vi "Login.vi"(9 "connection reference":T1, 10 "ACCOUNT:":string, 11 "Permission":string[](array[string])) -> (2 "OK":bool=TRUE, 3 "ACCOUNT:  2":string)   [LabVIEW 2015]
uses:
  <vilib>/addons/database/Connection.llb/Conn ObjectReference.ctl
  <vilib>/addons/database/_DB Variant To Data/Database Variant To Data.xnode
  <vilib>/addons/database/NI_Database_API.lvlib
  <vilib>/addons/database/Connection.llb/DB Tools Open Connec (String).vi
panel:
  out "Account Data":string[][](array[string])
  in  "Cancel":bool
  in  "Login":bool
  in  "PASSWORD:":string
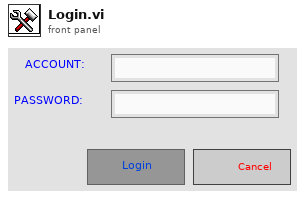
[diagram p1: front panel]
types:
  T1 = typedef "NI_Database_API.lvlib/Conn ObjectReference.ctl" = refnum<k1>
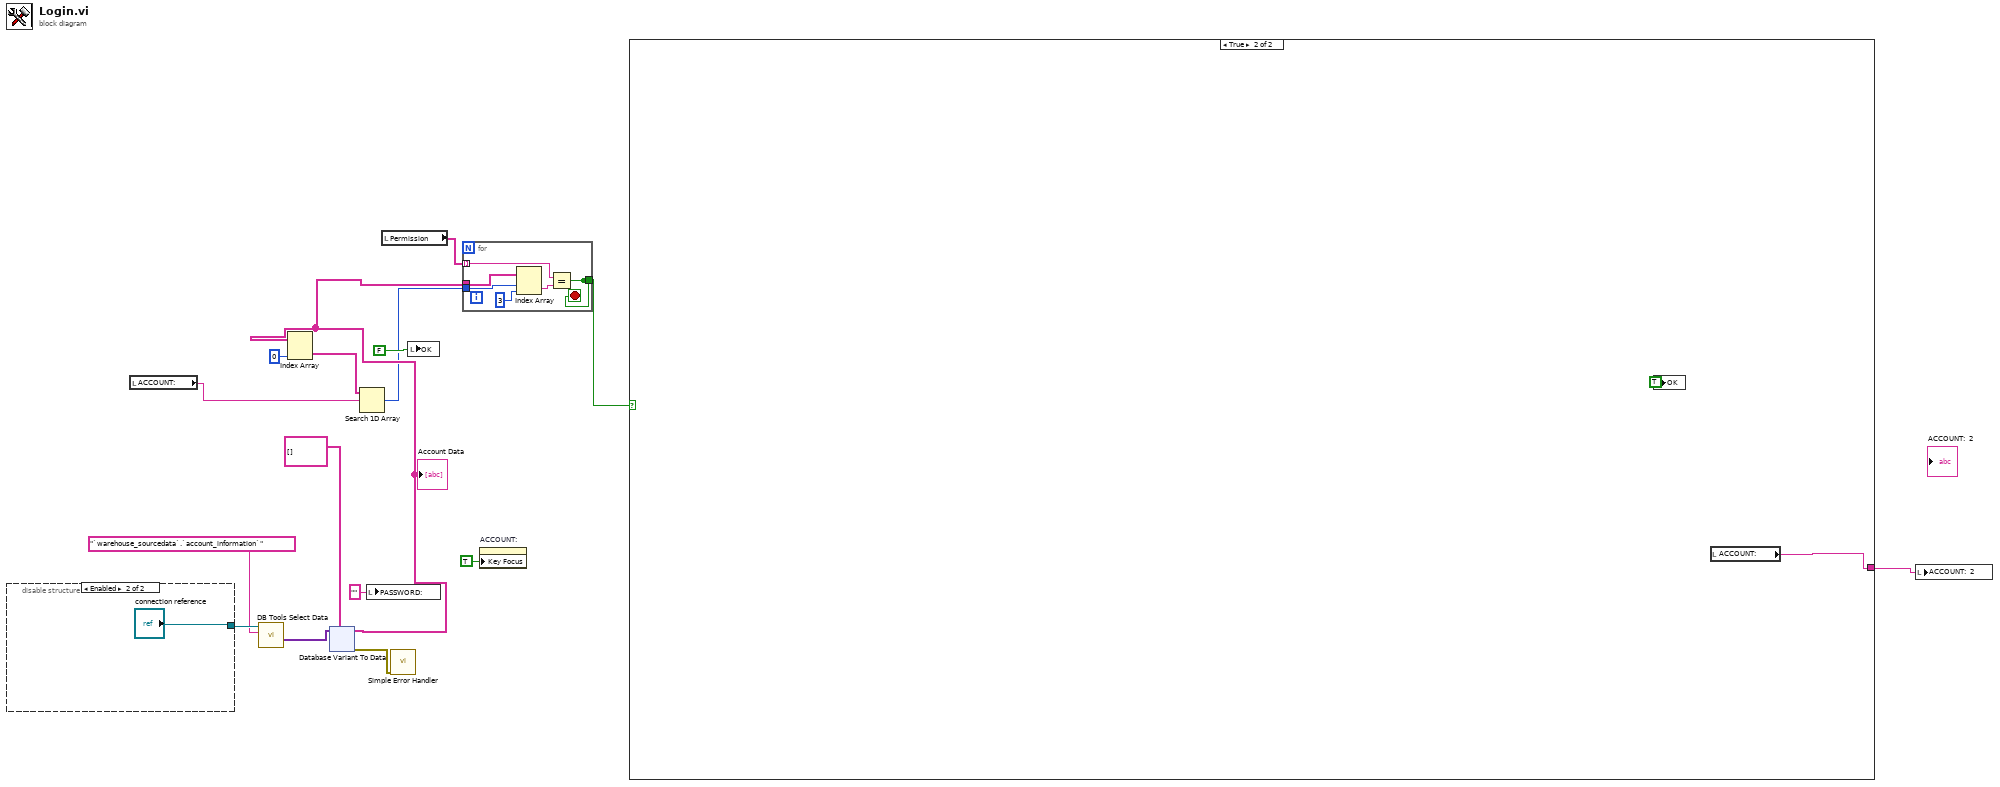
[diagram p0: block diagram]
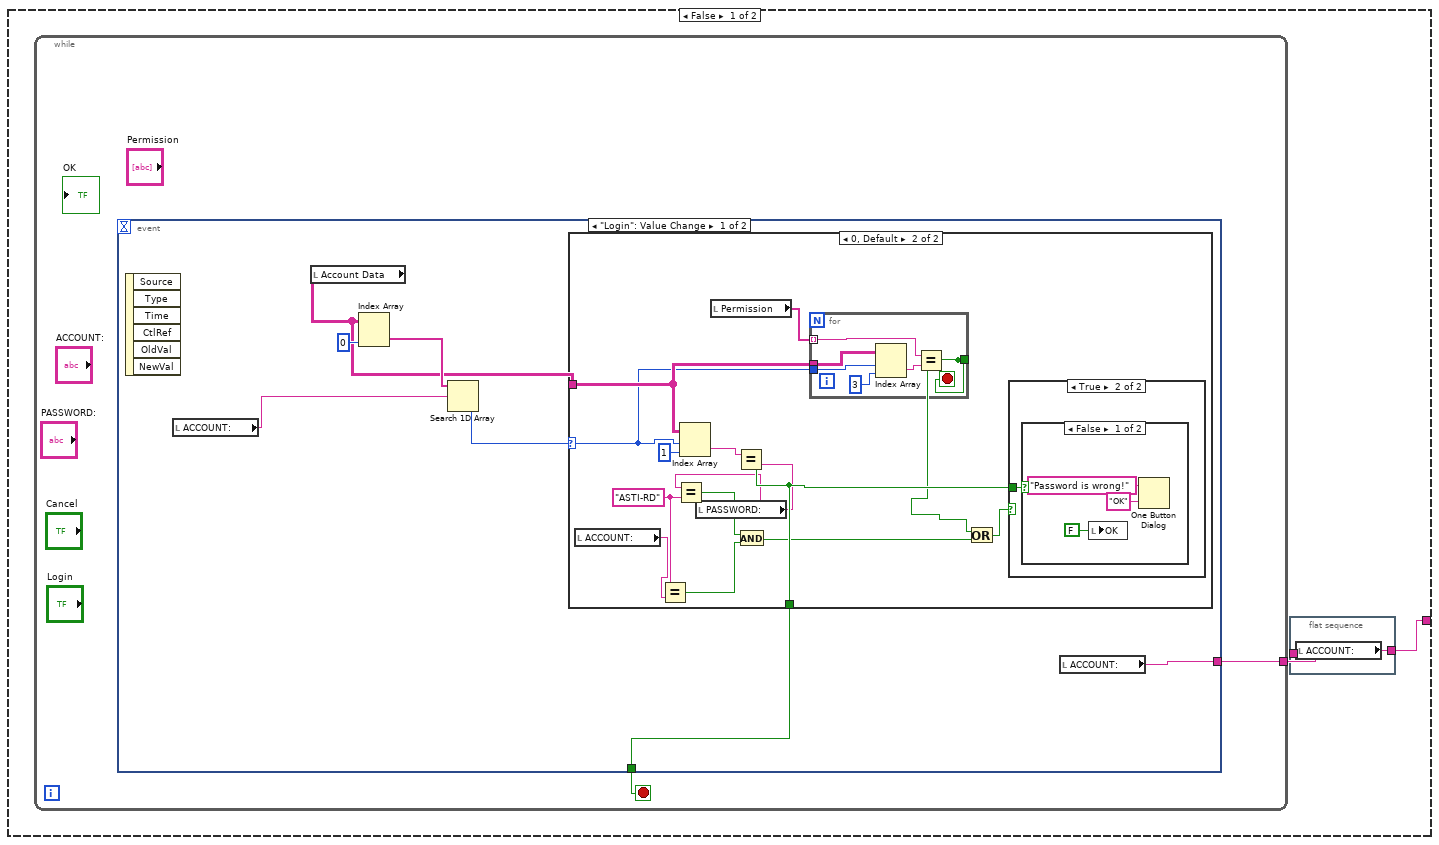
[diagram p2: hidden frame]
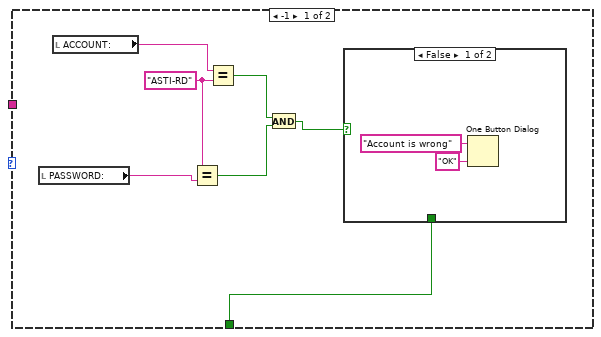
[diagram p3: hidden frame]
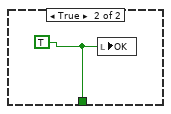
[diagram p4: hidden frame]
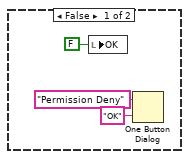
[diagram p5: hidden frame]
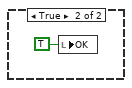
[diagram p6: hidden frame]
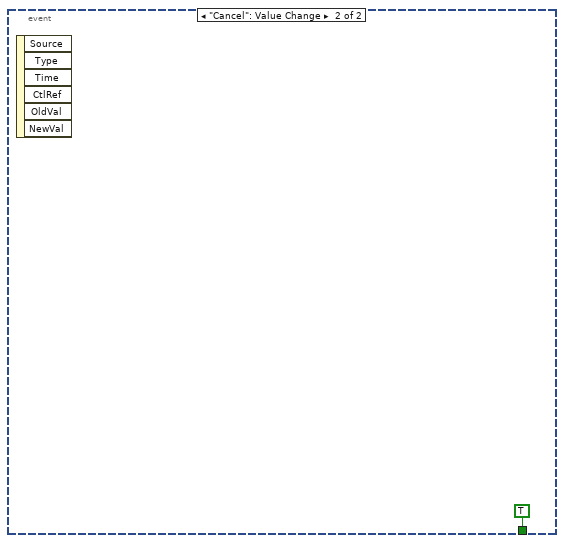
[diagram p7: hidden frame]
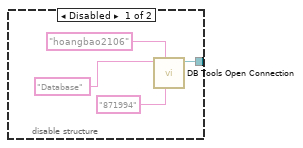
[diagram p8: hidden frame]
diagram:
  n1 = disable-structure shown="Enabled" {
    disable-tunnel: [w17 "connection reference"] -> w14
    frame Disabled {
      n2 = call-poly <vilib>:"DB Tools Open Connection.vi"("password"="871994" ("userID"), "userID"="hoangbao2106", "connection information"="Database" ("userID")) -> ("connection reference"=w17:T1)  [unwired: 5 in, 1 out]
    }
    frame Enabled {
    }
  }
  n3 = local read "ACCOUNT:"() -> (w7:string)
  n4 = call <vilib>:"DB Tools Select Data.vi"("table"="`warehouse_sourcedata`.`account_information`" ("userID"), "connection reference"=w14) -> ("data"=w12:variant[][])  [unwired: 4 in, 2 out]
  n5 = xnode "Database Variant To Data"("database variant"=w12, "type"=string[][] []) -> ("data"=w5:string[][], "error out"=w10:errorcluster)  [unwired: 1 in]
  "Account Data" <- w5
  n6 = Index Array(array=w5, index (col)=0 ("disabled index (col)")) -> (element=w9:string[])  [unwired: 1 in]
  n7 = Search 1D Array(1D array=w9, element=w7) -> (index of element=w4:i32)  [unwired: 1 in]
  n8 = local write "PASSWORD:"("" ("PASSWORD:")) -> ()
  n9 = local read "Permission"() -> (w6:string[])
  n10 = call <vilib>:"Simple Error Handler.vi"("error in (no error)"=w10) -> ()  [unwired: 4 in, 5 out]
  n11 = local write "OK"(FALSE) -> ()
  n12 = for {
    tunnel: w5 -> [w27]
    tunnel: w4 -> [w25]
    tunnel: w6 -> [w23] mode=indexing
    tunnel: [w22] -> w3
    stop <- w22 stop-if-true
    n13 = Index Array(array=w27, index (row)=w25, index (col)=3 ("index")) -> (element=w24:string)
    n14 = Equal?(x=w23, y=w24) -> (x = y?=w22:bool)
  }
  n15 = property on="ACCOUNT:" class="Str"("Key Focus"=TRUE) -> ()  [unwired: 2 in, 2 out]
  n16 = case shown="True" w3 {
    tunnel: [w28 w79] -> w2
    frame False {
      n17 = while {
        tunnel: [w31] -> w29
        stop <- w32 stop-if-true
        n18 = event shown="[0] \"Login\": Value Change" {
          selector: _ -> [_ _]
          dyn-events: _ -> [_ _]
          timeout: _ -> [_ _]
          tunnel: [w36 TRUE] -> w32
          tunnel: [w33 _] -> w31
          event "Login": Value Change {
            n19 = event-data() -> ()  [unwired: 1 in, 6 out]
            n20 = local read "ACCOUNT:"() -> (w37:string)
            n21 = local read "Account Data"() -> (w34:string[][])
            n22 = Index Array(array=w34, index (col)=0 ("disabled index (col)")) -> (element=w38:string[])  [unwired: 1 in]
            n23 = Search 1D Array(1D array=w38, element=w37) -> (index of element=w35:i32)  [unwired: 1 in]
            n24 = case shown="0, Default" w35 {
              selector: w35 -> [_ w58]
              tunnel: w34 -> [_ w59]
              tunnel: [w40 w60] -> w36
              frame -1 {
                w44 = "ASTI-RD" ("y")
                n25 = local read "PASSWORD:"() -> (w45:string)
                n26 = local read "ACCOUNT:"() -> (w46:string)
                n27 = Equal?(x=w44, y=w45) -> (x = y?=w42:bool)
                n28 = Equal?(x=w46, y=w44) -> (x = y?=w43:bool)
                n29 = And(x=w43, y=w42) -> (x .and. y?=w41:bool)
                n30 = case shown="False" w41 {
                  tunnel: [_ w49] -> w40
                  frame False {
                    n31 = One Button Dialog(message="Account is wrong", button name ("OK")="OK") -> ()  [unwired: 1 out]
                  }
                  frame True {
                    w49 = TRUE
                    n32 = local write "OK"(w49) -> ()
                  }
                }
              }
              frame 0, Default {
                w57 = "ASTI-RD" ("y")
                n33 = local read "ACCOUNT:"() -> (w51:string)
                n34 = Equal?(x=w57, y=w51) -> (x = y?=w55:bool)
                n35 = Index Array(array=w59, index (row)=w58, index (col)=1 ("disabled index (col)")) -> (element=w62:string)
                n36 = local read "PASSWORD:"() -> (w52:string)
                n37 = Equal?(x=w52, y=w57) -> (x = y?=w56:bool)
                n38 = local read "Permission"() -> (w61:string[])
                n39 = Equal?(x=w62, y=w52) -> (x = y?=w60:bool)
                n40 = And(x=w56, y=w55) -> (x .and. y?=w54:bool)
                n41 = for {
                  tunnel: w59 -> [w69]
                  tunnel: w58 -> [w67]
                  tunnel: w61 -> [w65] mode=indexing
                  tunnel: [w64] -> w50
                  stop <- w64 stop-if-true
                  n42 = Index Array(array=w69, index (row)=w67, index (col)=3 ("index")) -> (element=w66:string)
                  n43 = Equal?(x=w65, y=w66) -> (x = y?=w64:bool)
                }
                n44 = Or(x=w50, y=w54) -> (x .or. y?=w53:bool)
                n45 = case shown="True" w53 {
                  tunnel: w60 -> [_ w73]
                  frame False {
                    n46 = local write "OK"(FALSE ("OK")) -> ()
                    n47 = One Button Dialog(message="Permission Deny", button name ("OK")="OK") -> ()  [unwired: 1 out]
                  }
                  frame True {
                    n48 = case shown="False" w73 {
                      frame False {
                        n49 = local write "OK"(FALSE ("OK")) -> ()
                        n50 = One Button Dialog(message="Password is wrong!", button name ("OK")="OK") -> ()  [unwired: 1 out]
                      }
                      frame True {
                        n51 = local write "OK"(TRUE ("OK")) -> ()
                      }
                    }
                  }
                }
              }
            }
            n52 = local read "ACCOUNT:"() -> (w33:string)
          }
          event "Cancel": Value Change {
            n53 = event-data() -> ()  [unwired: 1 in, 6 out]
          }
        }
      }
      n54 = flat-sequence {
        tunnel: w29 -> [_]
        tunnel: [w30] -> w28
        frame #0 {
          n55 = local read "ACCOUNT:"() -> (w30:string)
        }
      }
    }
    frame True {
      n56 = local write "OK"(TRUE ("OK")) -> ()
      n57 = local read "ACCOUNT:"() -> (w79:string)
    }
  }
  n58 = local write "ACCOUNT:  2"(w2) -> ()
